vi "Simple writing on screen.vi"() -> ()   [LabVIEW 2014, in "Arduino LiquidCrystal Wrapper.lvlib"]
uses:
  <vilib>/Aledyne-TSXperts/Arduino Compatible Compiler for LabVIEW/addons/Arduino LiquidCrystal Wrapper/Arduino LiquidCrystal Wrapper.lvlib
panel:
  out "Bytes count read":u16
  out "Error Out":errorcluster
  in  "Error In":errorcluster
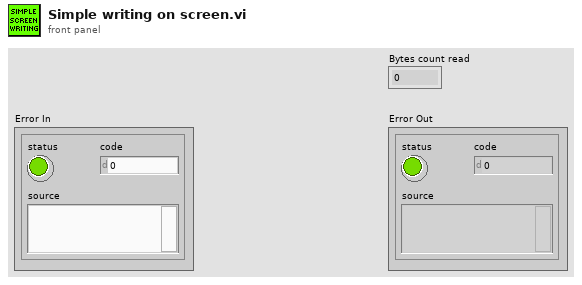
[diagram p1: front panel]
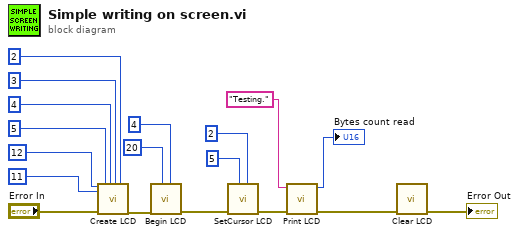
[diagram p0: block diagram]
diagram:
  n1 = call <vilib>:"Create LCD.vi"("rs"=u8 12, "enable"=u8 11, "Error In"="Error In", "d4"=u8 5, "d5"=u8 4, "d6"=u8 3, "d7"=u8 2) -> ("Error Out"=w10:errorcluster)  [unwired: 12 in]
  n2 = call <vilib>:"Begin LCD.vi"("rows"=u8 4, "cols"=u8 20, "Error In"=w10) -> ("Error Out"=w18:errorcluster)  [unwired: 8 in]
  n3 = call <vilib>:"SetCursor LCD.vi"("row"=u8 2, "col"=u8 5, "Error In"=w18) -> ("Error Out"=w7:errorcluster)  [unwired: 8 in]
  n4 = call <vilib>:"Print LCD.vi"("Error In"=w7, "text"="Testing.") -> ("Error Out"=w1:errorcluster, "Bytes count read"=→"Bytes count read":u16)  [unwired: 8 in]
  n5 = call <vilib>:"Clear LCD.vi"("Error In"=w1) -> ("Error Out"=→"Error Out":errorcluster)  [unwired: 8 in]
